vi "Mach_Interpolation.vi"() -> ()   [LabVIEW 2016]
uses:
  <vilib>/Utility/file.llb/Read Delimited Spreadsheet (DBL).vi
panel:
  out "Math_OUT":dbl[](array[numeric])
  out "XY Graph 4":cluster{"Y":dbl[], "Y":dbl[]}[](graph)
  out "XY Graph 3":cluster{"Y":dbl[], "Y":dbl[]}[](graph)
  out "XY Graph 2":cluster{"Y":dbl[], "Y":dbl[]}[](graph)
  out "XY Graph":cluster{"Y":dbl[], "Y":dbl[]}[](graph)
  out "size(s)":i32[](array[numeric])
  out "all rows":dbl[][](array[numeric]) format="%.9g"
  # "Math                                   G1                                       G2                                        G3                                          G4"
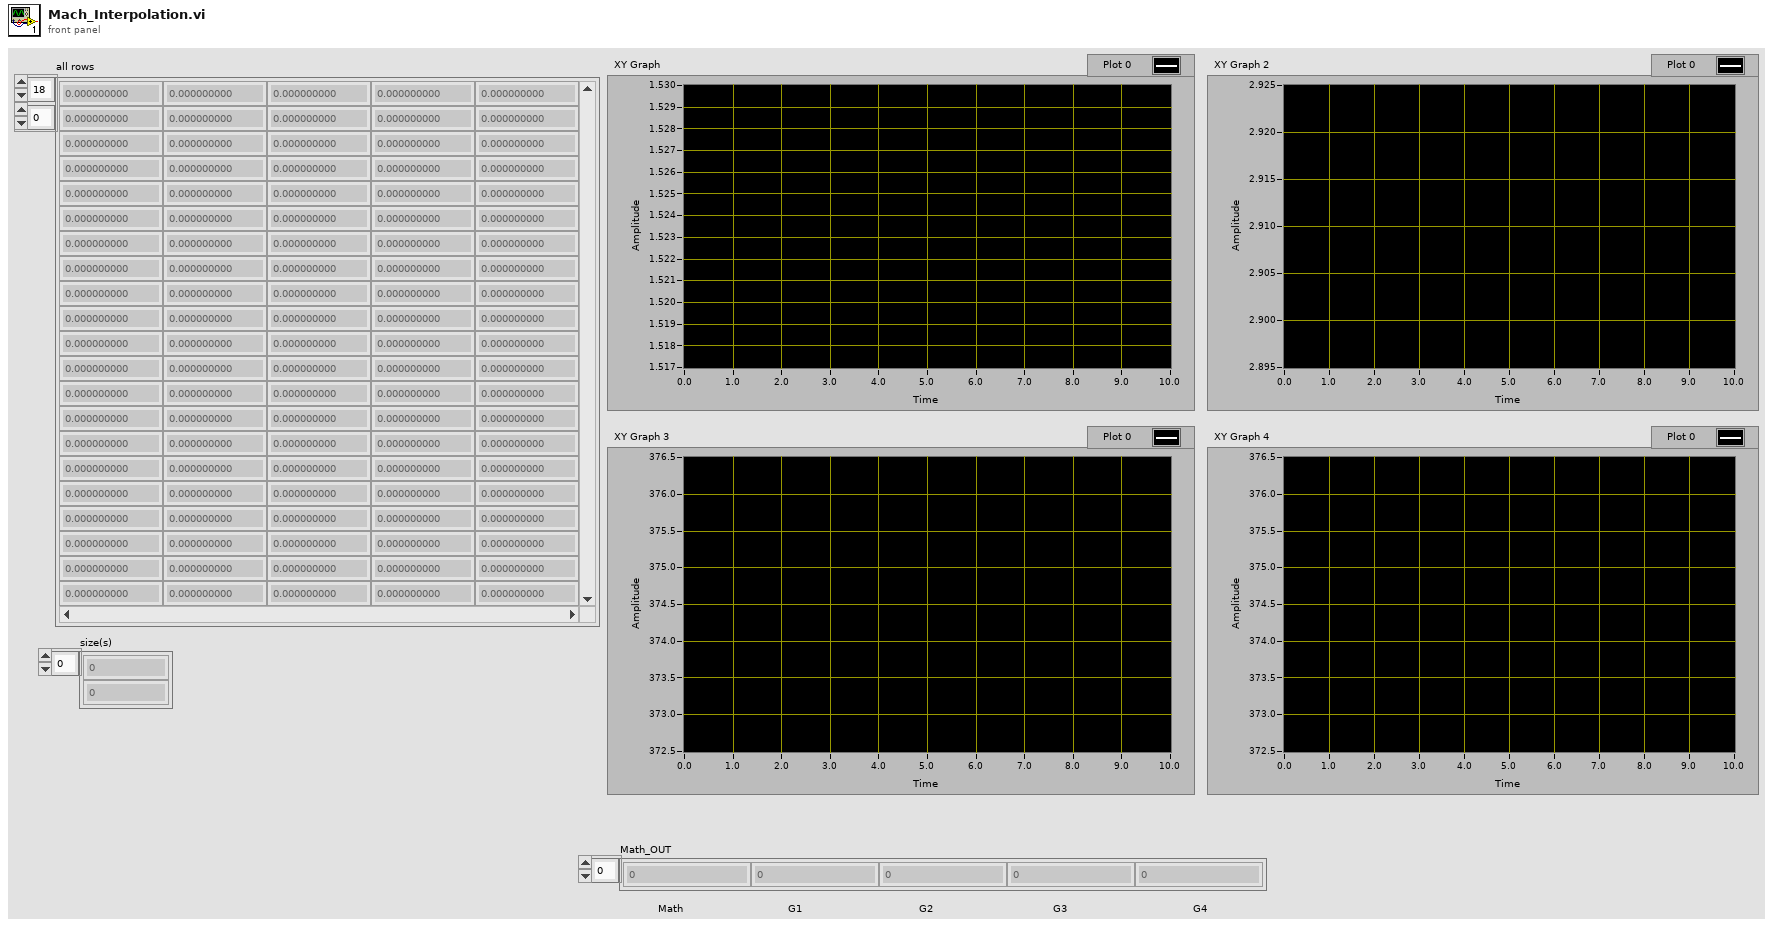
[diagram p1: front panel]
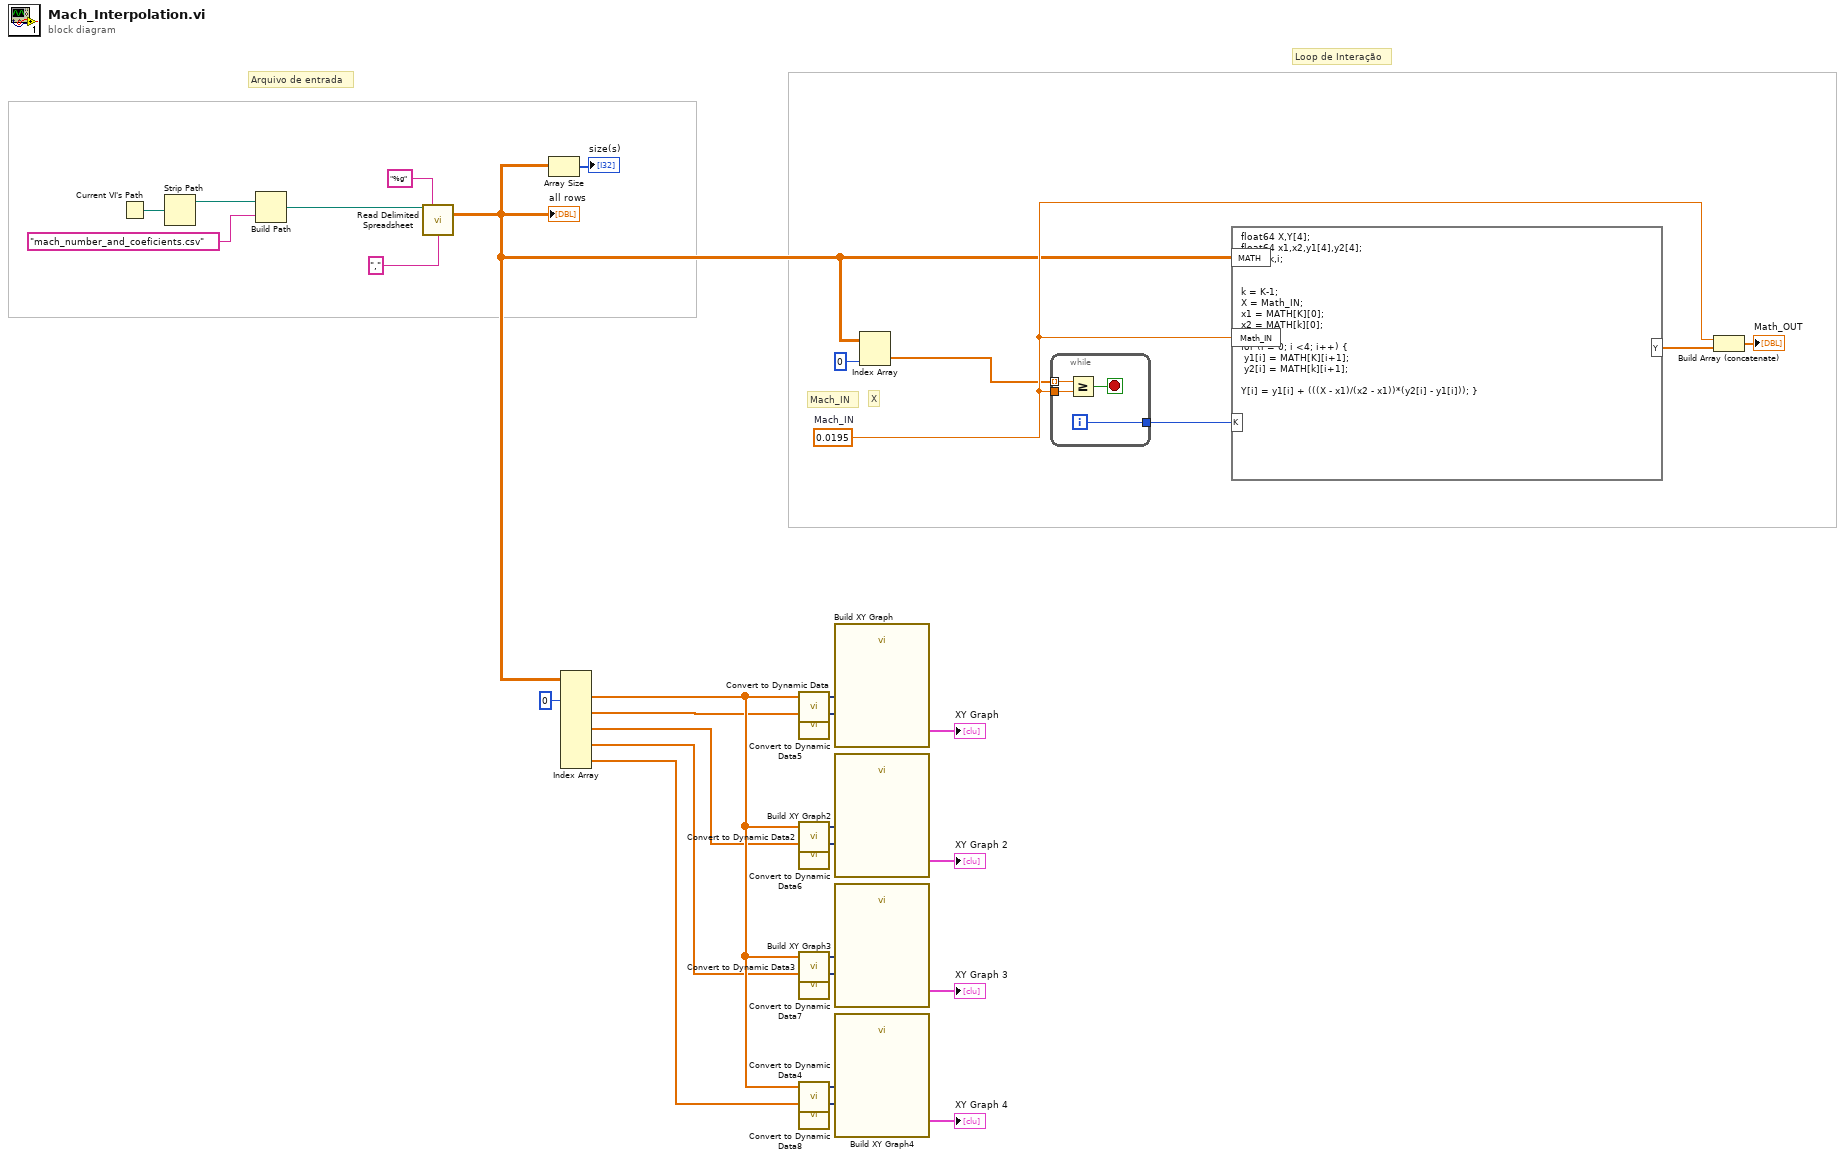
[diagram p0: block diagram]
diagram:
  w6 = 0.0195  # Mach_IN
  # "Arquivo de entrada"
  # "Loop de Interação"
  # "X"
  # "Mach_IN"
  n1 = Current VI's Path() -> (path=w32:path)
  n2 = Strip Path(path=w32) -> (stripped path=w31:path)  [unwired: 1 out]
  n3 = Build Path(base path=w31, name or relative path="mach_number_and_coeficients.csv") -> (appended path=w29:path)
  n4 = call-poly <vilib>:"Read Delimited Spreadsheet.vi"("file path (dialog if empty)"=w29, "format (%.3f)"="%g", "delimiter (\\t)"="," ("delimiter (\\t)")) -> ("all rows"=w3:dbl[][])  [unwired: 7 in, 5 out]
  "all rows" <- w3
  n5 = Array Size(array=w3) -> (size(s)=→"size(s)":i32[])
  n6 = Index Array(array=w3, index (col) #1=0 ("disabled index (col)")) -> (element #1=w12:dbl[], element #2=w11:dbl[], element #3=w10:dbl[], element #4=w9:dbl[], element #5=w8:dbl[])  [unwired: 9 in]
  n7 = call "Convert to Dynamic Data"("Array"=w12) -> ("Dynamic Data Type"=w20:dynamicdata)  [unwired: 3 in]
  n8 = call "Convert to Dynamic Data5"("Array"=w11) -> ("Dynamic Data Type"=w16:dynamicdata)  [unwired: 3 in]
  n9 = call "Convert to Dynamic Data2"("Array"=w12) -> ("Dynamic Data Type"=w19:dynamicdata)  [unwired: 3 in]
  n10 = call "Convert to Dynamic Data6"("Array"=w10) -> ("Dynamic Data Type"=w15:dynamicdata)  [unwired: 3 in]
  n11 = call "Convert to Dynamic Data3"("Array"=w12) -> ("Dynamic Data Type"=w18:dynamicdata)  [unwired: 3 in]
  n12 = call "Convert to Dynamic Data7"("Array"=w9) -> ("Dynamic Data Type"=w14:dynamicdata)  [unwired: 3 in]
  n13 = call "Convert to Dynamic Data4"("Array"=w12) -> ("Dynamic Data Type"=w17:dynamicdata)  [unwired: 3 in]
  n14 = call "Convert to Dynamic Data8"("Array"=w8) -> ("Dynamic Data Type"=w13:dynamicdata)  [unwired: 3 in]
  n15 = call "Build XY Graph"("Y Input"=w16, "X Input"=w20) -> ("XY Graph"=→"XY Graph":cluster{"X":dbl[], "Y":dbl[]}[])  [unwired: 8 in, 1 out]
  n16 = call "Build XY Graph2"("Y Input"=w15, "X Input"=w19) -> ("XY Graph"=→"XY Graph 2":cluster{"X":dbl[], "Y":dbl[]}[])  [unwired: 8 in, 1 out]
  n17 = call "Build XY Graph3"("Y Input"=w14, "X Input"=w18) -> ("XY Graph"=→"XY Graph 3":cluster{"X":dbl[], "Y":dbl[]}[])  [unwired: 8 in, 1 out]
  n18 = call "Build XY Graph4"("Y Input"=w13, "X Input"=w17) -> ("XY Graph"=→"XY Graph 4":cluster{"X":dbl[], "Y":dbl[]}[])  [unwired: 8 in, 1 out]
  n19 = Index Array(array=w3, index (col)=0 ("disabled index (col)")) -> (element=w1:dbl[])  [unwired: 1 in]
  n20 = while {
    tunnel: w1 -> [w35] mode=indexing
    tunnel: w6 -> [w33]
    tunnel: [w34] -> w7
    i -> [w34]
    stop <- w36 stop-if-true
    n21 = Greater Or Equal?(x=w35, y=w33) -> (x >= y?=w36:bool)
  }
  n22 = formula code="float64 X,Y[4];\nfloat64 x1,x2,y1[4],y2[4];\nint32 k,i;\n\n\nk = K-1;\nX = Math_IN;\nx1 = MATH[K][0];\nx2 = MATH[k][0];\n\nfor (i = 0; i <4; i++) {\n y1[i] = MATH[K][i+1]; \n y2[i] = MATH[k][i+1]; \n\nY[i] = y1[i] + (((X - x1)/(x2 - x1))*(y2[i] - y1[i])); }"("K"=w7, "MATH"=w3, "Math_IN"=w6) -> ("Y"=w5:dbl[])
  n23 = Build Array (concatenate)(w6, w5) -> (→"Math_OUT":dbl[])
